vi "Database.File.Move.vi"(8 "error in (no error)":errorcluster, 10 "FileName":string, 11 "Data in":T1={"Status"={"Run"=FALSE, "Handle"=0, "ConnTS"=timestamp(0 s since 1904-01-01), "DbTime"=timestamp(0 s since 1904-01-01), "DbTimeCode"=0.0, "DbTimeOffset"=0.0}, "Sets"={"Enable"=FALSE, "R/W"=FALSE, "LogDebug"=FALSE, "ConnString"="", "ProductionLine"="", "SystemName1"="T075", "SystemName2"=""}, "Results"={"Service"=FALSE, "Ref"="", "Serial"="", "ID"={"processId"=0, "systemId"=0, "processStepId"=0, "wabcoPartId"=0}, "P"={"c_id"="", "productId"="", "processId"=0, "statusId"=0, "startTime"="", "endTime"=""}, "PS"={"c_id"="", "processResultId"="", "processStepId"=0, "statusId"=0, "operatorId"=0, "startTime"="", "endTime"=""}, "TS"=[]}, "Variant"={"Found"=FALSE, "Ref"="", "ID"={"processId"=0, "systemId"=0, "processStepId"=0, "wabcoPartId"=0}, "PP"=[], "TS"=[]}} {"Variant"."TS"."TV"."minimum" format="%#.3f"; "Variant"."TS"."TV"."maximum" format="%#.3f"; "Variant"."TS"."TP"."value" format="%#.3f"}) -> (0 "error out":errorcluster, 3 "Data out":T1={"Status"={"Run"=FALSE, "Handle"=0, "ConnTS"=timestamp(0 s since 1904-01-01), "DbTime"=timestamp(0 s since 1904-01-01), "DbTimeCode"=0.0, "DbTimeOffset"=0.0}, "Sets"={"Enable"=FALSE, "R/W"=FALSE, "LogDebug"=FALSE, "ConnString"="", "ProductionLine"="", "SystemName1"="T075", "SystemName2"=""}, "Results"={"Service"=FALSE, "Ref"="", "Serial"="", "ID"={"processId"=0, "systemId"=0, "processStepId"=0, "wabcoPartId"=0}, "P"={"c_id"="", "productId"="", "processId"=0, "statusId"=0, "startTime"="", "endTime"=""}, "PS"={"c_id"="", "processResultId"="", "processStepId"=0, "statusId"=0, "operatorId"=0, "startTime"="", "endTime"=""}, "TS"=[]}, "Variant"={"Found"=FALSE, "Ref"="", "ID"={"processId"=0, "systemId"=0, "processStepId"=0, "wabcoPartId"=0}, "PP"=[], "TS"=[]}} {"Variant"."TS"."TV"."minimum" format="%#.3f"; "Variant"."TS"."TV"."maximum" format="%#.3f"; "Variant"."TS"."TP"."value" format="%#.3f"})   [LabVIEW 2016]
uses:
  Database.Main.Data.ctl
  Database.Main.Data.Status.ctl
  Database.Main.Data.Sets.ctl
  Database.Main.Data.Results.ctl
  ProdaNG/Controls/ProdaNG.Identification.ctl
  ProdaNG/Controls/ProdaNG.ProcessResult.ctl
  ProdaNG/Controls/ProdaNG.ProcessStepResult.ctl
  ProdaNG/Controls/ProdaNG.TestStepResult.ctl
  ProdaNG/Controls/ProdaNG.TestValueResult.ctl
  Database.Main.Data.Variant.ctl
  ProdaNG/Controls/ProdaNG.ProcessStepParam.ctl
  ProdaNG/Controls/ProdaNG.TestStep.ctl
  ProdaNG/Controls/ProdaNG.TestStepParam.ctl
  ProdaNG/Controls/ProdaNG.TestValue.ctl
  tools/EventLog/EventLog.EventSource.ctl
  tools/Translator/Translator.Message.ctl
  tools/EventLog/EventLog.New(single).vi
  Global/ApplicationGlobal.vi
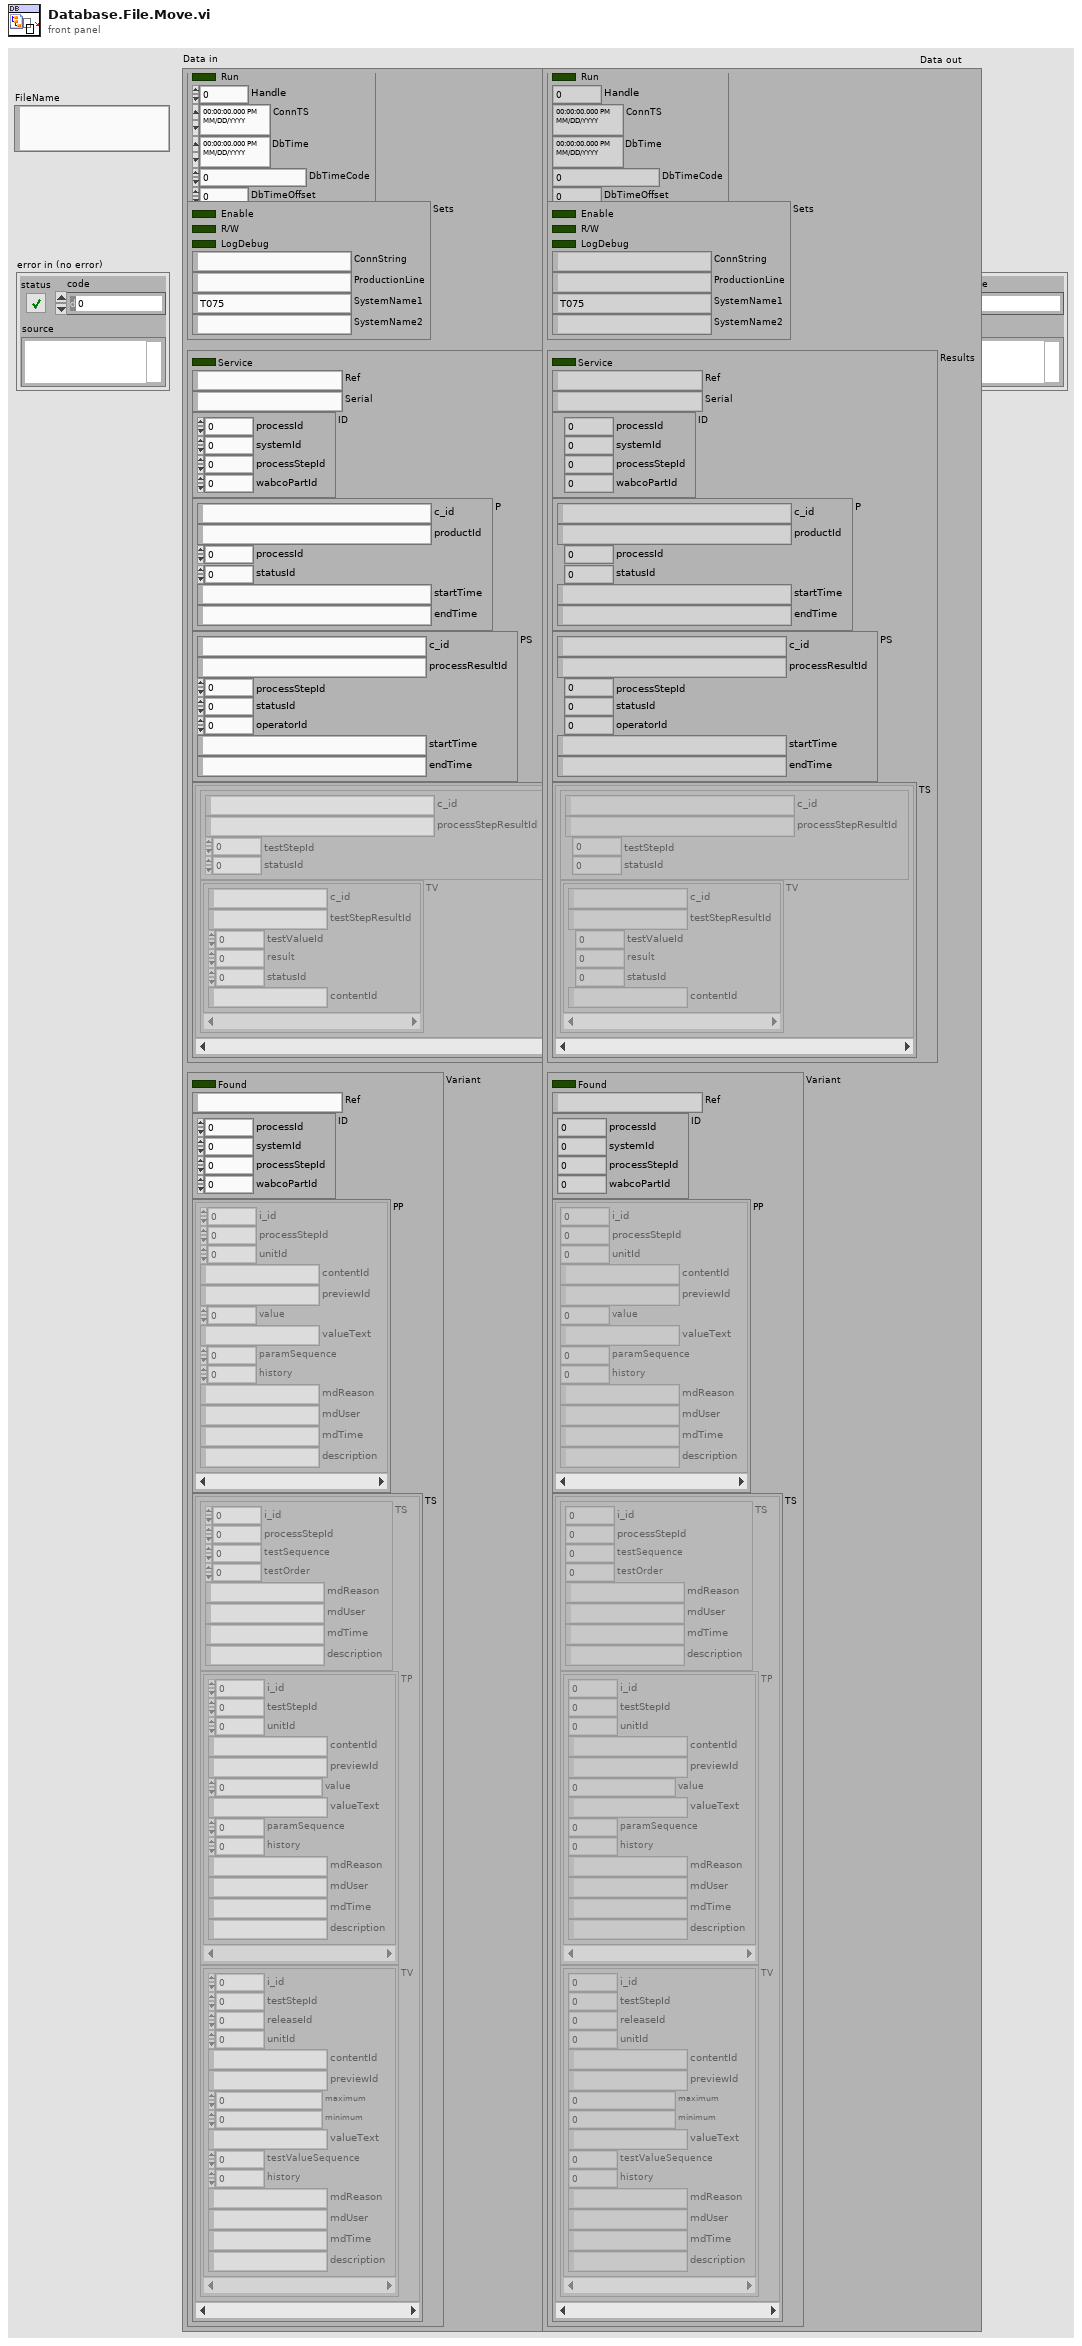
[diagram p1: front panel]
types:
  T1 = typedef "Database.Main.Data.ctl" = cluster{"Status":T2, "Sets":T3, "Results":T4, "Variant":T10}
  T2 = typedef "Database.Main.Data.Status.ctl" = cluster{"Run":bool, "Handle":i32, "ConnTS":timestamp, "DbTime":timestamp, "DbTimeCode":dbl, "DbTimeOffset":dbl}
  T3 = typedef "Database.Main.Data.Sets.ctl" = cluster{"Enable":bool, "R/W":bool, "LogDebug":bool, "ConnString":string, "ProductionLine":string, "SystemName1":string, "SystemName2":string}
  T4 = typedef "Database.Main.Data.Results.ctl" = cluster{"Service":bool, "Ref":string, "Serial":string, "ID":T5, "P":T6, "PS":T7, "TS":cluster{"TS":T8, "TV":T9[]}[]}
  T5 = typedef "ProdaNG.Identification.ctl" = cluster{"processId":i32, "systemId":i32, "processStepId":i32, "wabcoPartId":i32}
  T6 = typedef "ProdaNG.ProcessResult.ctl" = cluster{"c_id":string, "productId":string, "processId":i32, "statusId":i32, "startTime":string, "endTime":string}
  T7 = typedef "ProdaNG.ProcessStepResult.ctl" = cluster{"c_id":string, "processResultId":string, "processStepId":i32, "statusId":i32, "operatorId":i32, "startTime":string, "endTime":string}
  T8 = typedef "ProdaNG.TestStepResult.ctl" = cluster{"c_id":string, "processStepResultId":string, "testStepId":i32, "statusId":i32}
  T9 = typedef "ProdaNG.TestValueResult.ctl" = cluster{"c_id":string, "testStepResultId":string, "testValueId":i32, "result":dbl, "statusId":i32, "contentId":string}
  T10 = typedef "Database.Main.Data.Variant.ctl" = cluster{"Found":bool, "Ref":string, "ID":T5, "PP":T11[], "TS":cluster{"TS":T12, "TP":T13[], "TV":T14[]}[]}
  T11 = typedef "ProdaNG.ProcessStepParam.ctl" = cluster{"i_id":i32, "processStepId":i32, "unitId":i32, "contentId":string, "previewId":string, "value":dbl, "valueText":string, "paramSequence":i32, "history":i32, "mdReason":string, "mdUser":string, "mdTime":string, "description":string}
  T12 = typedef "ProdaNG.TestStep.ctl" = cluster{"i_id":i32, "processStepId":i32, "testSequence":i32, "testOrder":i32, "mdReason":string, "mdUser":string, "mdTime":string, "description":string}
  T13 = typedef "ProdaNG.TestStepParam.ctl" = cluster{"i_id":i32, "testStepId":i32, "unitId":i32, "contentId":string, "previewId":string, "value":dbl, "valueText":string, "paramSequence":i32, "history":i32, "mdReason":string, "mdUser":string, "mdTime":string, "description":string}
  T14 = typedef "ProdaNG.TestValue.ctl" = cluster{"i_id":i32, "testStepId":i32, "releaseId":i32, "unitId":i32, "contentId":string, "previewId":string, "maximum":dbl, "minimum":dbl, "valueText":string, "testValueSequence":i32, "history":i32, "mdReason":string, "mdUser":string, "mdTime":string, "description":string}
  T15 = typedef "Translator.Message.ctl" = enum16{"-", "Event confirmed", "Log out", "Log in", "Shutdown", "Cancel", "Start", "Begin time", "End time", "Duration", "Service Mode", "Ignore Results", "Serial Format", "On", "Off", "OK", "NOK", "NOK %s", "Home", "Work", "Close", "Open", "In progress...", "Missing", "Empty", "Hardware failure", "Initial", "Default", "Total", "Out of range", "Free disk space is below 1GB - contact technician", "Error %d >> %s", "Error %d >> %s >> %s", "Msg %d >> %s", "Laser msg %d %s", "Laser cmd error %s %d", "Laser cmd failed %s", "Laser cmd warning %s", "Laser disconnected", "Laser status %s", "Laser already started", "Laser job unkonwn %s", "Laser job missing %s", "Laser job select failure %s", "Unable to start laser printing (%s)", "Unable to stop laser printing (%s)", "Laser marking aborted", "Laser marking timeout", "Unable to reset Laser Interlock (%s)", "Unable to trigger Laser. Laser not ready (%s)", "Laser job '%s' coordinates not configured", "Starting %s", "Quitting %s", "Configured", "Initializing", "Quitting", "Loading", "Loaded %d results", "Loaded %d events", "Running", "Stopped", "Summary", "Laser", "Do you want to continue?", "Do you want to delete the configuration?", "The configuration is being used by an order. Unable to delete!", "Press confirm button", "Station is not based. Do you want to exit?", "Station requires changeover. Do you want to run the test?", "Test options are not set as default. Do you want to continue?", "Formatting of WabcoNo is disabled. Do you want to continue?", "Product not detected. Do you want to continue?", "Product scan failed. Do you want to continue?", "Calibration", "Log out?", "System", "All", "IDLE", "Translating...%s", "Not found", "Alarm %s", "Run", "Skip", "Abort", "Repeat", "Please wait...", "Database disconnected", "Database disconnected - changeover disabled!", "Login to database successful", "Login to database failed: %d; %s", "Unable to check the product status of reference %d - database disconnected", "Unable to set the product status of reference %d - database disconnected", "Variant file backup %s", "Read variant (%s)", "Result", "Station armed!", "Station requires changeover!", "Select reference number...", "EMERGENCY BUTTON - press Control button", "EMERGENCY DOOR - press Control button", "Resetting Emergency...", "Unable to reset safety circuit - Emergency Button pressed", "Unable to reset safety circuit - Emergency Side Door open", "Station not based", "Station based", "Station not empty", "Station basing...", "No order", "Press Start to begin new order", "Scanning new order", "Order NOK. Correct or scan again", "Order OK. Press Accept", "Order ready", "Revolver incorrect", "Fork incorrect", "Revolver missing", "Revolver empty", "Container missing", "Offline results", "Offline statistics", "Updating statistics %.1f %%", "DMC Configurator", "Door open", "Close the front door", "Press start button", "Done. Open the front door", "Running...", "Running...%.1f %%", "Pause %s", "Pause %s. NOK container missing", "Pause %s. OK container missing", "Pause %s. Revolver empty", "Pause %s. Revolver missing", "Pause %s. Revolver incorrect", "Pause %s. Fork missing", "Pause %s. Fork incorrect", "Pause %s. Too many failures", "Pause %s. Unloading failure", "Pause %s. One slot is not working", "Pause %s. Part order is done. Empty OK container", "Pause %s. Unable to move product to slot", "Pause %s. Unable to move back product pusher", "Pause %s. Unable to lift product", "Pause %s. Unable to move back product lifter", "Pause %s. Unable to move product arm to Work", "Pause %s. Unable to move product arm to NOK", "Pause %s. Unable to move product arm to OK", "Pause %s. Unable to unsuck the NOK product", "Pause %s. Unable to drop the NOK product", "Pause %s. Product OK missing", "Pause %s. Unable to unsuck the OK product", "Pause %s. Unable to drop the OK product", "Stopping...", "File '%s' is missing", "File '%s' is broken", "File '%s' is running", "Log file started (%s)", "Log file ended (%s)", "Log file stopped (%s)", "Log file ignored (%s)", "Log file exported (%s)", "Log file export failed (%s)", "Wrong serial number in log file", "Wrong reference number in log file", "Test steps are missing", "%s = %.3f", "Process param '%s' not found in DB", "Process param '%s' wrong order", "Process param '%s' value %.3f out of limits (%.3f; %.3f)", "Step%d param '%s' not found in DB", "Step%d param '%s' wrong order", "Step%d param '%s' value %.3f out of limits (%.3f; %.3f)", "Step%d EV '%s' not found in DB", "Step%d EV '%s' wrong order", "\"%s\" not found in DB", "\"%s\" wrong order", "\"%s\" value %.3f out of limits (%.3f; %.3f)", "\"%s\" not found in software", "Process init (%s)", "Process started", "Process restarted", "Process run", "Process done", "Process done - remove OK container", "Process aborted", "Process aborted at work", "Process aborted at home", "Process error", "Process error at home", "Process error at work", "Process close", "Process pause", "Process continue", "Process door open", "Process door close", "Process pause at slot %s due to %s", "Select plate from the order to process", "Do you want to start the process?", "Do you want to continue the process?", "There is unfinished order. Do you want to put the new order?", "Product %s %d OK", "Product %s %d NOK", "Unable to unload the slot %s. Product missing in the slot", "Unable to unload the slot %s. Product already in the arm", "Unable to accept the product as OK. Product missing in slot %s", "Unable to accept the product as OK. Product could not drop into the container at slot %s", "Unable to accept the product as NOK. Product could not drop into the container at slot %s", "Scan failed. Error %s", "Scan failed. Scanner disconnected", "Scan failed. Wrong Wabco number %d, limit (%d,%d)", "Scan failed. Wrong serial number %d, limit (%d,%d)", "Scan failed. Wrong date %d, limit (%d,%d)", "Scan failed. Wrong product wabco number %d (expected %d)", "Scan failed. Wrong product serial number %d (expected > 0)", "Scan OK %s", "Scan failed. Unable to determine table position (%s)", "Scan failed. Timeout", "Tune failed. Scanner disconnected", "Tune failed. Timeout", "%s = %d", "%s = %d->%d", "Unable to set %s = %.2f - Air Pressure Inside off", "Unable to set digital output '%s' = %d", "Unable to activate air pressure inside - timeout", "Unable to activate air pressure inside - aborted", "Unable to switch on Air Main Valve - Air Pressure Inlet off", "Unable to switch on Air Main Valve - Door open", "Unable to switch off Air Main Valve - timeout", "Unable to switch off Air Main Valve - aborted", "Unable to rotate Table - timeout", "Unable to rotate Table - aborted", "Unable to rotate Table - Product Move not in Home position", "Unable to rotate Table - Air Pressure Inside off", "Unable to rotate Table - Product Lift A not in Home position", "Unable to rotate Table - Product Lift B not in Home position", "Unable to rotate Table - unlock before movement timeout", "Unable to rotate Table - lock after movement timeout", "Unable to move Table Lock to %s position - timeout", "Unable to move Table Lock to %s position - aborted", "Unable to move Table Lock to %s position - Air Pressure Inside off", "Unable to move Table Lock to %s position - Table not in position", "Unable to move Product Lift A to %s position - timeout", "Unable to move Product Lift B to %s position - timeout", "Unable to move Product Lift A to %s position - aborted", "Unable to move Product Lift B to %s position - aborted", "Unable to move Product Lift A to %s position - Air Pressure Inside off", "Unable to move Product Lift B to %s position - Air Pressure Inside off", "Unable to move Product Lift A to %s position - Table not locked", "Unable to move Product Lift B to %s position - Table not locked", "Unable to move Product Lift A to %s position - Product Arm not in Work position", "Unable to move Product Lift B to %s position - Product Arm not in Work position", "Unable to set Product Suction Gripper %s to %s - timeout", "Unable to set Product Suction Gripper %s to %s - aborted", "Unable to set Product Suction Gripper %s to %s - Air Pressure Inside off", "Unable to set Product Suction Gripper %s to %s - Table slot unkown", "Unable to move Product Arm to %s position - timeout", "Unable to move Product Arm to %s position - aborted", "Unable to move Product Arm to %s position - Air Pressure Inside off", "Unable to move Product Arm to %s position - Product Lift A not in Home position", "Unable to move Product Arm to %s position - Product Lift B not in Home position", "Unable to move Product to %s position - timeout", "Unable to move Product to %s position - aborted", "Unable to move Product to %s position - Air Pressure Inside off", "Unable to move Product to %s position - Table not in position"}
  T16 = typedef "EventLog.EventSource.ctl" = enum16{"All", "Gui", "Ref", "File", "Arch", "Seq", "CPX", "DB", "Laser", "Scan.P", "Scan.O"}
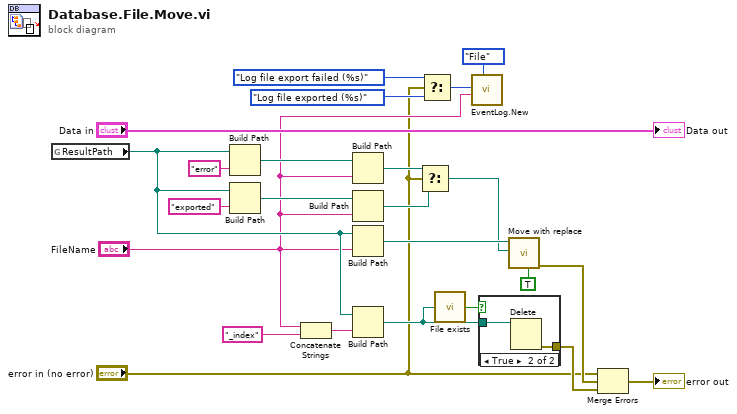
[diagram p0: block diagram]
diagram:
  n1 = global read "ApplicationGlobal.vi" "ResultPath"() -> (w17:path)
  n2 = Build Path(base path=w17, name or relative path="error") -> (appended path=w20:path)
  n3 = Build Path(base path=w17, name or relative path="exported") -> (appended path=w21:path)
  n4 = Concatenate Strings("FileName", "_index" ("string")) -> (w18:string)
  n5 = Build Path(base path=w20, name or relative path="FileName") -> (appended path=w15:path)
  n6 = Build Path(base path=w21, name or relative path="FileName") -> (appended path=w14:path)
  n7 = Build Path(base path=w17, name or relative path="FileName") -> (appended path=w16:path)
  n8 = Build Path(base path=w17, name or relative path=w18) -> (appended path=w11:path)
  n9 = Select(t=w15, s="error in (no error)", f=w14) -> (s? t:f=w13:path)
  n10 = Select(t=Translator.Message."Log file export failed (%s)" ("msg"), s="error in (no error)", f=Translator.Message."Log file exported (%s)" ("msg")) -> (s? t:f=w8:T15)
  n11 = call "File exists.vi"("file path"=w11) -> ("exists?"=w10:bool)  [unwired: 4 in]
  n12 = call-poly "EventLog.New.vi"("Source (All)"=EventLog.EventSource."File", "Arg"="FileName", "Message (-)"=w8) -> ()  [unwired: 7 in, 2 out]
  n13 = case shown="True" w10 {
    tunnel: w11 -> [_ w26]
    tunnel: [_ w25] -> w4
    frame False {
    }
    frame True {
      n14 = Delete(path (use dialog)=w26) -> (error out=w25:errorcluster)  [unwired: 4 in, 2 out]
    }
  }
  n15 = call "Move with replace.vi"("create parent dirs (F)"=TRUE, "destination path"=w13, "source path"=w16) -> ("error"=w3:errorcluster)  [unwired: 8 in]
  n16 = Merge Errors("error in (no error)", w3, w4) -> (→"error out":errorcluster)
  "Data out" <- "Data in"
